vi "Query Error Status.vi"(8 "error in (no error)":errorcluster, 11 "VISA resource name":refnum<visa-resource-name>) -> (0 "error out":errorcluster, 2 "Error Status Data Message":string, 3 "VISA resource name out":refnum<visa-resource-name>)   [LabVIEW 2020, in "Stanford Research 830.lvlib"]
doc: "Queries the Error Status register for the Error Data Register group. Essentially, it is used to observe possible invalid results."
uses:
  Stanford Research 830.lvlib
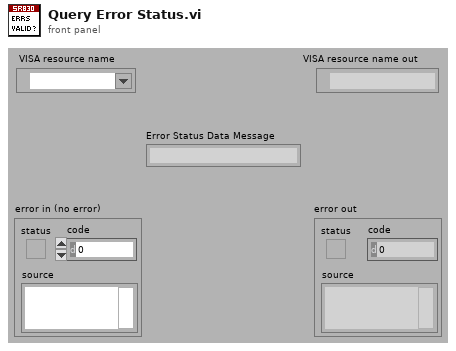
[diagram p1: front panel]
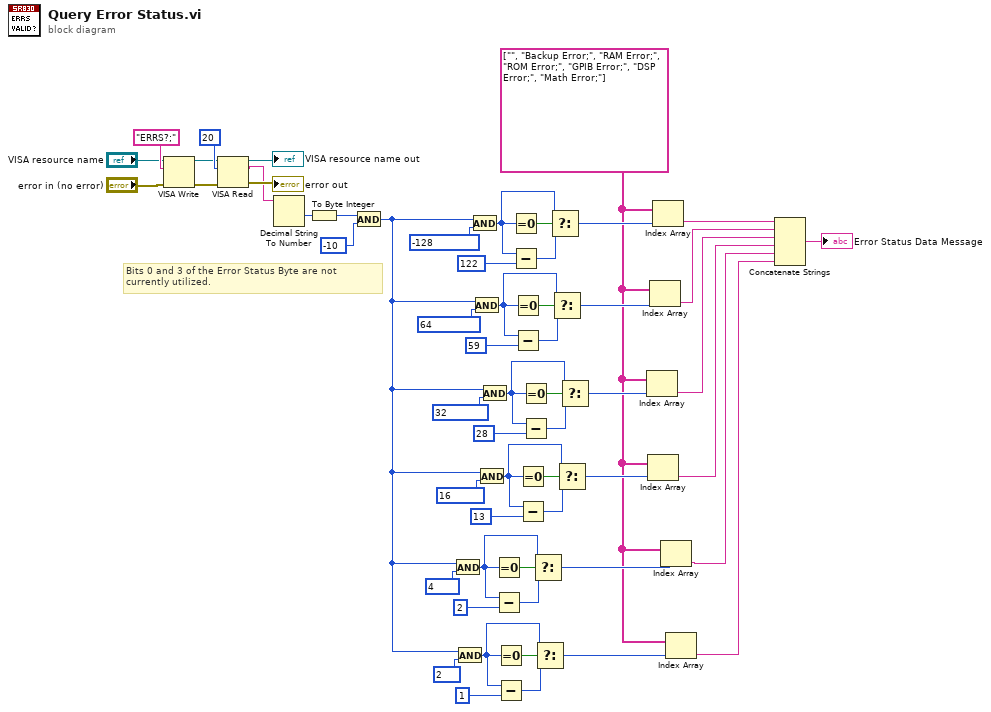
[diagram p0: block diagram]
diagram:
  w8 = string[] ["", "Backup Error;", "RAM Error;", "ROM Error;", "GPIB Error;", "DSP Error;", "Math Error;"]
  # "Bits 0 and 3 of the Error Status Byte are not currently utilized."
  n1 = VISA Write(VISA resource name="VISA resource name", write buffer="ERRS?;", error in (no error)="error in (no error)") -> (VISA resource name out=w54:refnum<visa-resource-name>, error out=w53:errorcluster)  [unwired: 1 out]
  n2 = VISA Read(VISA resource name=w54, byte count=u32 20, error in (no error)=w53) -> (VISA resource name out=→"VISA resource name out":refnum<visa-resource-name>, read buffer=w1:string, error out=→"error out":errorcluster)  [unwired: 1 out]
  n3 = Decimal String To Number(string=w1) -> (number=w57:i32)  [unwired: 2 in, 1 out]
  n4 = To Byte Integer(number=w57) -> (8bit integer=w44:i8)
  n5 = And(x=w44, y=i8 -10 ("value")) -> (x .and. y?=w4:i8)
  n6 = And(x=w4, y=i8 4) -> (x .and. y?=w17:i8)
  n7 = And(x=w4, y=i8 2) -> (x .and. y?=w10:i8)
  n8 = And(x=w4, y=i8 -128) -> (x .and. y?=w43:i8)
  n9 = And(x=w4, y=i8 64) -> (x .and. y?=w38:i8)
  n10 = And(x=w4, y=i8 16) -> (x .and. y?=w24:i8)
  n11 = And(x=w4, y=i8 32) -> (x .and. y?=w31:i8)
  n12 = Equal To 0?(x=w17) -> (x = 0?=w19:bool)
  n13 = Subtract(x=w17, y=i8 2) -> (x-y=w18:i8)
  n14 = Equal To 0?(x=w10) -> (x = 0?=w12:bool)
  n15 = Subtract(x=w10, y=i8 1) -> (x-y=w11:i8)
  n16 = Equal To 0?(x=w43) -> (x = 0?=w47:bool)
  n17 = Subtract(x=w43, y=i8 122) -> (x-y=w46:i8)
  n18 = Equal To 0?(x=w38) -> (x = 0?=w40:bool)
  n19 = Subtract(x=w38, y=i8 59) -> (x-y=w39:i8)
  n20 = Equal To 0?(x=w24) -> (x = 0?=w26:bool)
  n21 = Subtract(x=w24, y=i8 13) -> (x-y=w25:i8)
  n22 = Equal To 0?(x=w31) -> (x = 0?=w33:bool)
  n23 = Subtract(x=w31, y=i8 28) -> (x-y=w32:i8)
  n24 = Select(t=w17, s=w19, f=w18) -> (s? t:f=w15:i8)
  n25 = Select(t=w10, s=w12, f=w11) -> (s? t:f=w7:i8)
  n26 = Select(t=w43, s=w47, f=w46) -> (s? t:f=w45:i8)
  n27 = Select(t=w38, s=w40, f=w39) -> (s? t:f=w36:i8)
  n28 = Select(t=w24, s=w26, f=w25) -> (s? t:f=w22:i8)
  n29 = Select(t=w31, s=w33, f=w32) -> (s? t:f=w29:i8)
  n30 = Index Array(array=w8, index=w29) -> (element=w28:string)
  n31 = Index Array(array=w8, index=w22) -> (element=w21:string)
  n32 = Index Array(array=w8, index=w36) -> (element=w35:string)
  n33 = Index Array(array=w8, index=w45) -> (element=w48:string)
  n34 = Index Array(array=w8, index=w15) -> (element=w14:string)
  n35 = Index Array(array=w8, index=w7) -> (element=w6:string)
  n36 = Concatenate Strings(w48, w35, w28, w21, w14, w6) -> (→"Error Status Data Message":string)
